vi "Add XY (multiple).vi"(8 "error in (no error)":errorcluster, 9 "y":cluster{"X-array":dbl[], "Y-array":dbl[]}, 10 "x":cluster{"X-array":dbl[], "Y-array":dbl[]}, 11 "XY-data":cluster{"X-array":dbl[], "Y-array":dbl[]}[](array[cluster]) {"Y-array" format="%.2p"; "X-array" format="%.2p"}) -> (0 "error out":errorcluster, 3 "XY-data out":cluster{"X-array":dbl[], "Y-array":dbl[]}[](array[cluster]) {"Y-array" format="%.2p"; "X-array" format="%.2p"})   [LabVIEW 2019, in "xy_utilities.lvlib"]
doc: "Add <b>x</b>'s x array to the x array of <b>XY-data</b>\nAdd <b>y</b>'s y array to the y array of <b>XY-data</b>\n\nWire data to the data input to determine the polymorphic instance to use or manually select the instance."
uses:
  xy_utilities.lvlib
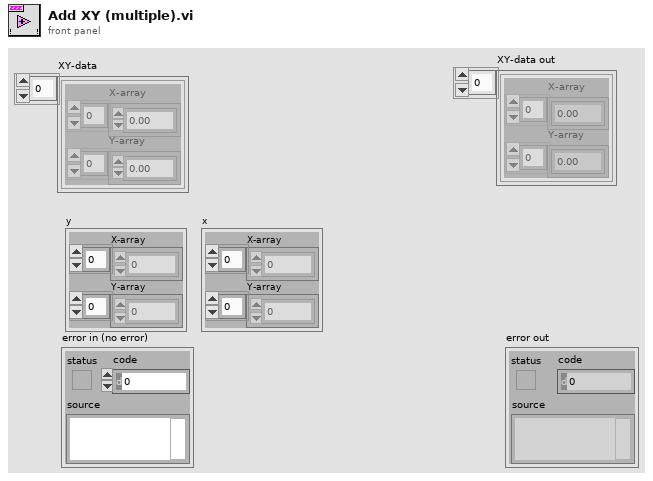
[diagram p1: front panel]
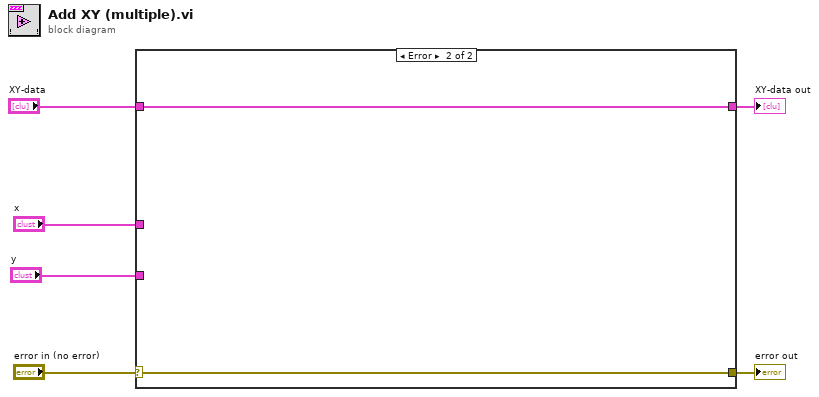
[diagram p0: block diagram]
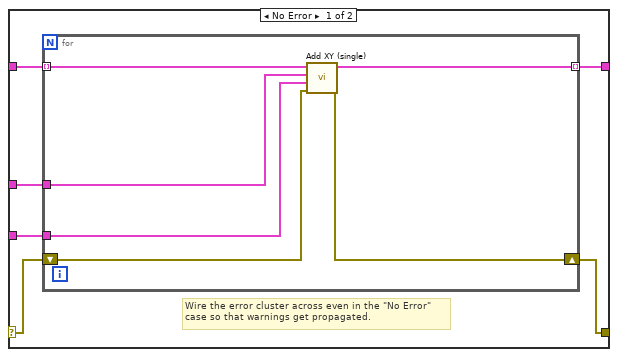
[diagram p2: hidden frame]
diagram:
  n1 = case shown="Error" "error in (no error)" {
    selector: "error in (no error)" -> [w8 w19]
    tunnel: [w7 w19] -> w1
    tunnel: "XY-data" -> [w12 w20]
    tunnel: [w11 w20] -> w4
    tunnel: "y" -> [w10 _]
    tunnel: "x" -> [w9 _]
    frame No Error {
      # "Wire the error cluster across even in the \"No Error\"\ncase so that warnings get propagated."
      n2 = for {
        tunnel: w12 -> [w16] mode=indexing
        tunnel: [w15] -> w11 mode=indexing
        tunnel: w10 -> [w18]
        tunnel: w9 -> [w13]
        shift-right: [w14] -> w7
        shift-left: w8 -> [w17]
        n3 = call "Add XY (single).vi"("error in (no error)"=w17, "y"=w18, "x"=w13, "XY-data"=w16) -> ("error out"=w14:errorcluster, "XY-data out"=w15:cluster{"X-array":dbl[], "Y-array":dbl[]})  [unwired: 6 in]
      }
    }
    frame Error {
    }
  }
  "error out" <- w1
  "XY-data out" <- w4
